vi "get Current.vi"(10 "current":dbl, 11 "devID":u32) -> (2 "current out":dbl, 3 "function return":i32)   [LabVIEW 2014, in "libchaos-driver-powersupply-labview.lvlib"]
doc: "int getCurrent(unsigned int devID,double*current);"
uses:
  libchaos-driver-powersupply-labview.lvlib
  chaos-i686-dynamic-release/lib/libchaos-driver-powersupply-labview.so
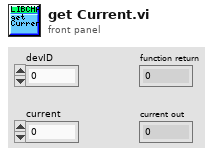
[diagram p1: front panel]
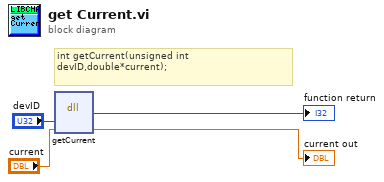
[diagram p0: block diagram]
diagram:
  # "int getCurrent(unsigned int devID,double*current);"
  n1 = dll-call lib="home/chaos/chaos_bundle/chaos-i686-dynamic-release/lib/libchaos-driver-powersupply-labview.*" fn="getCurrent"("devID"="devID", "current"="current") -> (→"function return":i32, "current"=→"current out":dbl)  [unwired: 4 in, 2 out]
